vi "Digital_Create.vi"(0 "reference in":refnum<class "Digital.lvclass">, 1 "Digits Total":dbl, 2 "Override size":cluster{"Width":i16, "Height":i16}, 3 "Digits Precision":dbl, 5 "error in (no error)":errorcluster) -> (14 "reference out":refnum<class "Digital.lvclass">, 19 "error out":errorcluster)   [LabVIEW 2019, in "Digital.lvclass"]
uses:
  Digital.lvclass
  C:/Users/Taylor.Hillegeist/OneDrive - Ultra/LabVIEW/Pgui2/Pgui_Obj_class/Pgui_Obj.lvclass
  Pgui_Obj_class/Pgui_Obj.lvclass
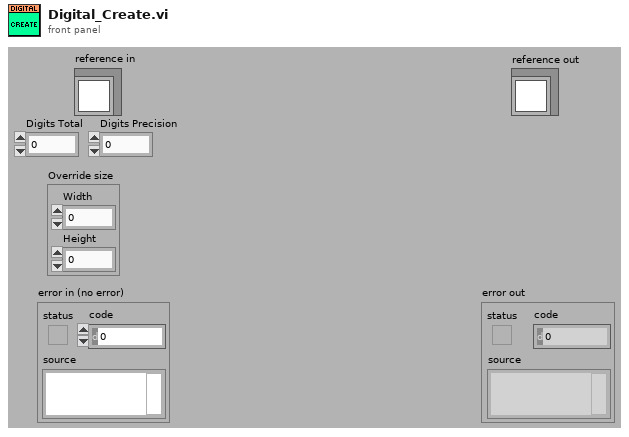
[diagram p1: front panel]
types:
  T1 = typedef "Digital.lvclass/ObjectAttributes.ctl" = cluster{"Override size":cluster{"Width":i16, "Height":i16}, "Value":dbl, "Digits Total":dbl, "Digits Precision":dbl}
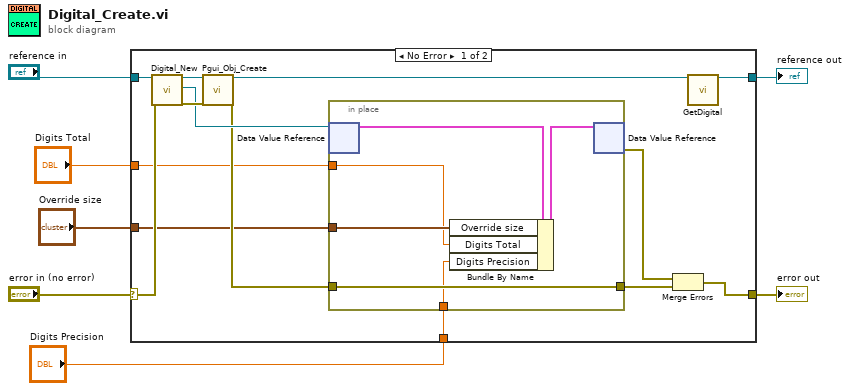
[diagram p0: block diagram]
diagram:
  n1 = case shown="No Error" "error in (no error)" {
    selector: "error in (no error)" -> [w20 w29]
    tunnel: [w18 w29] -> w6
    tunnel: "reference in" -> [w21 w28]
    tunnel: [w10 w28] -> w4
    tunnel: "Override size" -> [w12 _]
    tunnel: "Digits Total" -> [w9 _]
    tunnel: "Digits Precision" -> [w8 _]
    frame No Error {
      n2 = call "Digital_New.vi"("reference in"=w21, "error in (no error)"=w20) -> ("reference out"=w17:refnum<class "Digital.lvclass">, "DVRRefOut"=w15:refnum<data-value>, "error out"=w16:errorcluster)  [unwired: 14 in, 1 out]
      n3 = call "Pgui_Obj_Create.vi"("reference in"=w17, "error in (no error)"=w16) -> ("reference out"=w11:refnum<class "Digital.lvclass">, "error out"=w14:errorcluster)  [unwired: 16 in]
      n4 = in-place {
        in-place-border: w14 -> [w25]
        in-place-border: [w25] -> w13
        in-place-border: w12 -> [w24]
        in-place-border: w9 -> [w23]
        in-place-border: w8 -> [w22]
        n5 = in-place-dvr #1(w15) -> (w26:T1)  [unwired: 1 out]
        n6 = Bundle By Name(cluster=w26, "Override size"=w24, "Digits Total"=w23, "Digits Precision"=w22) -> (w27:T1)
        n7 = in-place-dvr #1(w27) -> (w19:errorcluster)  [unwired: 1 out]
      }
      n8 = Merge Errors(w19, w13) -> (w18:errorcluster)
      n9 = call-dynamic "GetDigital.vi"("reference in"=w11) -> ("reference out"=w10:refnum<class "Digital.lvclass">)  [unwired: 17 in, 1 out]
    }
    frame Error {
    }
  }
  "error out" <- w6
  "reference out" <- w4
